vi "HorizontalSetUp.vi"(0 "ActXDSO In":refnum<k7>, 1 "Sampling Rate":u16(ring)=5, 2 "Delay (micsec)":dbl format="%.3f", 3 "error in":errorcluster, 4 "rf points":i32=2000) -> (5 "ActXDSO Out":refnum<k7>, 6 "error out":errorcluster)   [LabVIEW 2022 SP3]
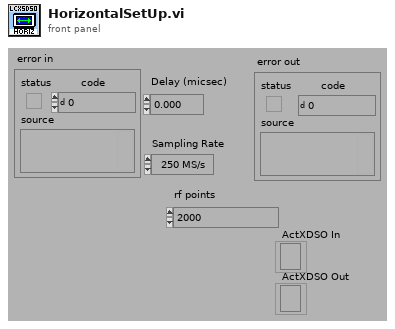
[diagram p1: front panel]
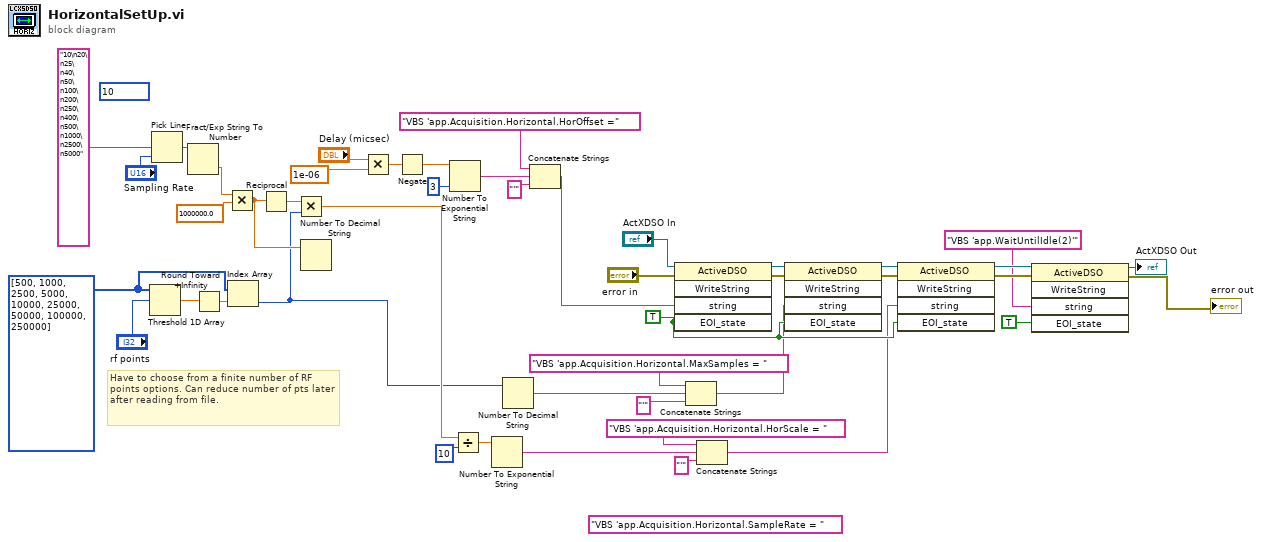
[diagram p0: block diagram]
diagram:
  w22 = TRUE
  (unwired) "VBS 'app.Acquisition.Horizontal.SampleRate = "
  (unwired) u16 10 ("Sampling Rate")
  w38 = i32[] [500, 1000, 2500, 5000, 10000, 25000, 50000, 100000, 250000]
  # "Have to choose from a finite number of RF points options. Can reduce number of pts later after reading from file."
  n1 = Threshold 1D Array(2:"rf points", 3:w38) -> (0:w40:dbl)  [unwired: 1 out]
  n2 = Pick Line(multi-line string="10\n20\n25\n40\n50\n100\n200\n250\n400\n500\n1000\n2500\n5000", line index="Sampling Rate") -> (output string=w44:string)  [unwired: 1 out]
  n3 = Fract/Exp String To Number(string=w44) -> (number=w43:dbl)  [unwired: 4 out]
  n4 = Round Toward +Infinity(x=w40) -> (ceil(x): smallest int >= x=w39:dbl)
  n5 = Multiply(x=w43, y=1000000.0) -> (x*y=w30:dbl)
  n6 = Index Array(array=w38, index=w39) -> (element=w28:i32)
  n7 = Reciprocal(x=w30) -> (1/x=w31:dbl)
  n8 = Multiply(x=w31, y=w28) -> (x*y=w35:dbl)
  n9 = Number To Decimal String(number=w30) -> ()  [unwired: 2 out]
  n10 = Multiply(x="Delay (micsec)", y=1e-06) -> (x*y=w34:dbl)
  n11 = Negate(x=w34) -> (-x=w13:dbl)
  n12 = Number To Exponential String(number=w13, precision (6)=3) -> (E-format string=w16:string)  [unwired: 2 out]
  n13 = Divide(x=w35, y=10) -> (x/y=w26:dbl)
  n14 = Number To Exponential String(number=w26) -> (E-format string=w5:string)  [unwired: 3 out]
  n15 = Number To Decimal String(number=w28) -> (decimal integer string=w3:string)  [unwired: 1 out]
  n16 = Concatenate Strings("VBS 'app.Acquisition.Horizontal.HorOffset =", w16, "'") -> (w15:string)
  n17 = invoke class="ActiveDSO" method="WriteString"(reference="ActXDSO In", error in="error in", "string"=w15, "EOI_state"=w22) -> (reference out=w21:refnum<k7>, error out=w23:errorcluster)  [unwired: 1 in, 3 out]
  n18 = Concatenate Strings("VBS 'app.Acquisition.Horizontal.MaxSamples = ", w3, "'") -> (w2:string)
  n19 = Concatenate Strings("VBS 'app.Acquisition.Horizontal.HorScale = ", w5, "'") -> (w1:string)
  n20 = invoke class="ActiveDSO" method="WriteString"(reference=w21, error in=w23, "string"=w2, "EOI_state"=w22) -> (reference out=w24:refnum<k7>, error out=w25:errorcluster)  [unwired: 1 in, 3 out]
  n21 = invoke class="ActiveDSO" method="WriteString"(reference=w24, error in=w25, "string"=w1, "EOI_state"=w22) -> (reference out=w11:refnum<k7>, error out=w10:errorcluster)  [unwired: 1 in, 3 out]
  n22 = invoke class="ActiveDSO" method="WriteString"(reference=w11, error in=w10, "string"="VBS 'app.WaitUntilIdle(2)'", "EOI_state"=TRUE) -> (reference out=→"ActXDSO Out":refnum<k7>, error out=→"error out":errorcluster)  [unwired: 1 in, 3 out]
